vi "MPU_Stick_Event_Counter.vi"(6 "Initialize ?":bool, 8 "error in (no error)":errorcluster, 9 "Event Name":string, 10 "Event count limits":i32[](array[numeric]), 11 "Event names":string[](array[string])) -> (0 "error out":errorcluster, 2 "Event occured":bool, 3 "Events":T1[](array[typedef]))   [LabVIEW 2017]
uses:
  Controls/MPU_Stick_Event.ctl
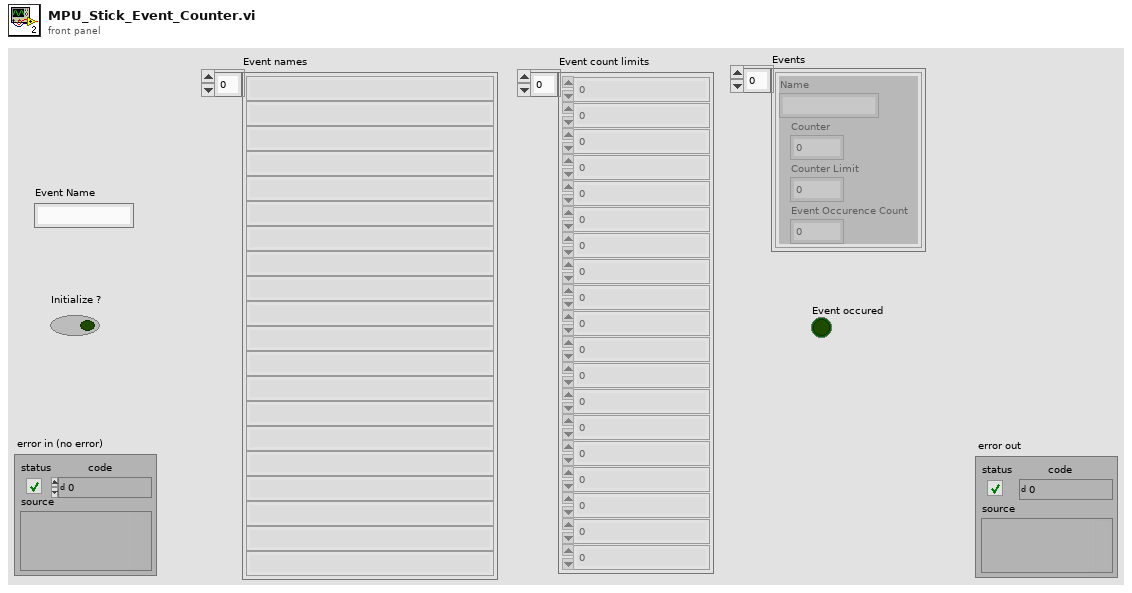
[diagram p1: front panel]
types:
  T1 = typedef "MPU_Stick_Event.ctl" = cluster{"Name":string, "Counter":i32, "Counter Limit":i32, "Event Occurence Count":i32}
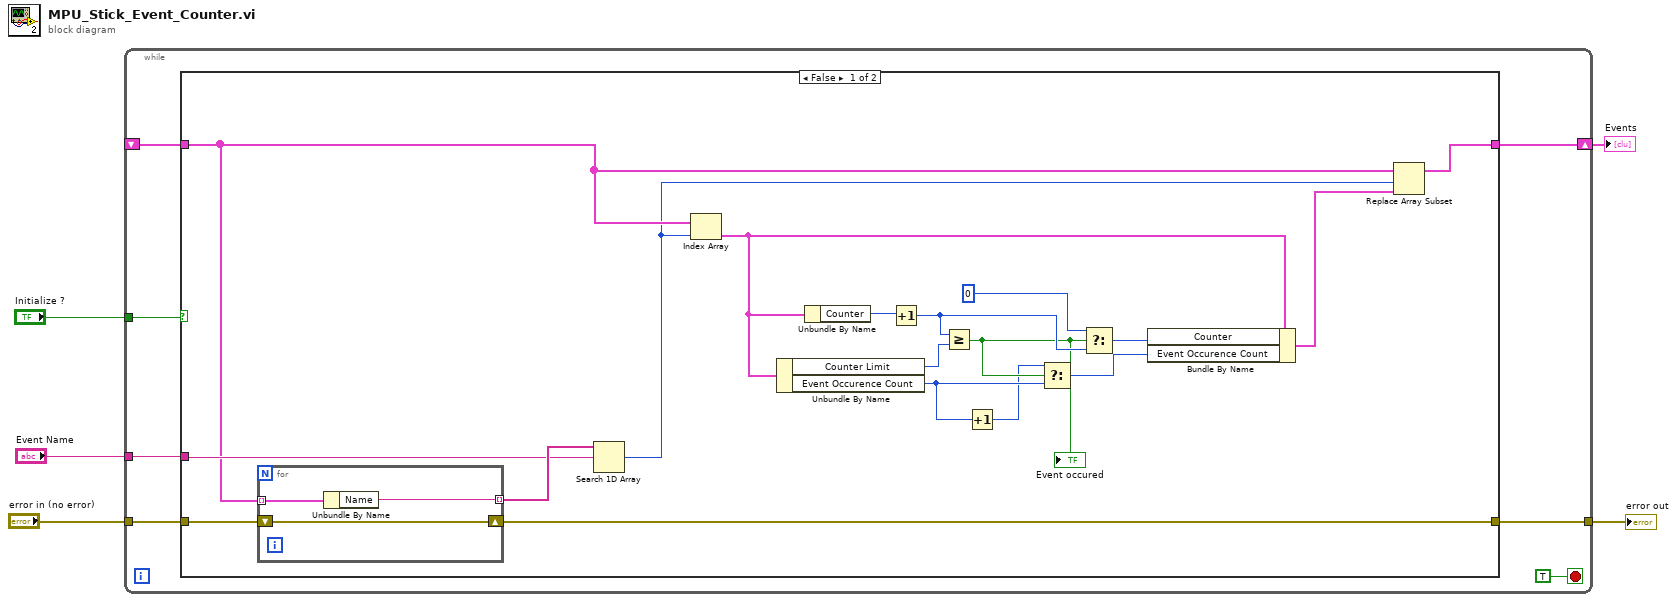
[diagram p0: block diagram]
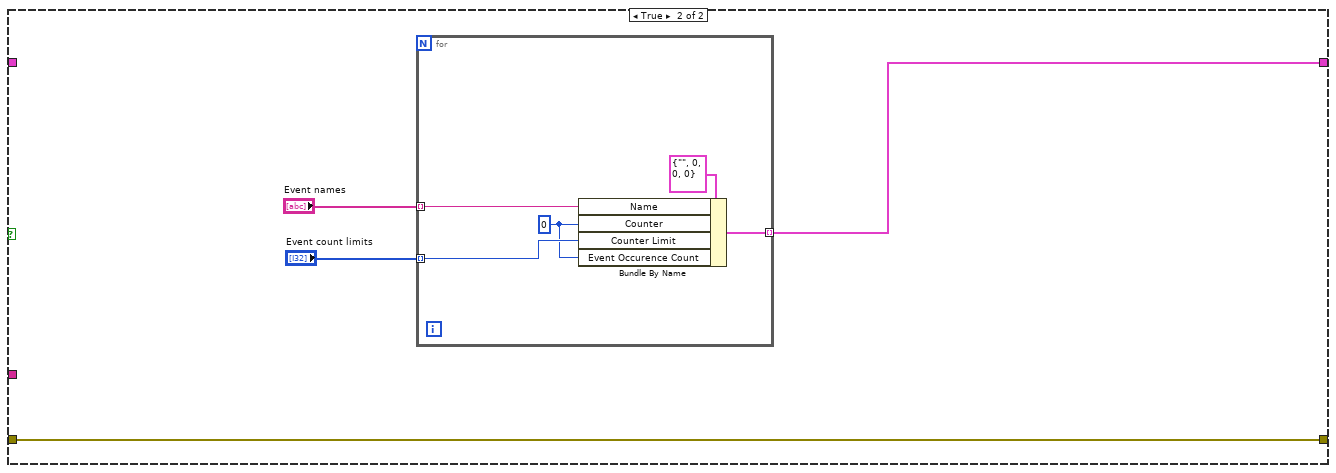
[diagram p2: hidden frame]
diagram:
  n1 = while {
    tunnel: "error in (no error)" -> [w11]
    tunnel: [w10] -> w4
    tunnel: "Initialize ?" -> [w9]
    shift-right: [w8] -> w1
    shift-left: _ -> [w7]
    tunnel: "Event Name" -> [w6]
    stop <- TRUE stop-if-true
    n2 = case shown="False" w9 {
      tunnel: w11 -> [w30 w37]
      tunnel: [w21 w37] -> w10
      tunnel: [w17 w34] -> w8
      tunnel: w7 -> [w20 _]
      tunnel: w6 -> [w28 _]
      frame False {
        n3 = for {
          shift-right: [w33] -> w21
          shift-left: w30 -> [w33]
          tunnel: w20 -> [w32] mode=indexing
          tunnel: [w31] -> w29 mode=indexing
          n4 = Unbundle By Name(w32) -> ("Name"=w31:string)
        }
        n5 = Search 1D Array(1D array=w29, element=w28) -> (index of element=w19:i32)  [unwired: 1 in]
        n6 = Index Array(array=w20, index=w19) -> (element=w23:T1)
        n7 = Unbundle By Name(w23) -> ("Counter Limit"=w26:i32, "Event Occurence Count"=w14:i32)
        n8 = Unbundle By Name(w23) -> ("Counter"=w27:i32)
        n9 = Increment(x=w27) -> (x+1=w25:i32)
        n10 = Greater Or Equal?(x=w25, y=w26) -> (x >= y?=w15:bool)
        "Event occured" <- w15
        n11 = Increment(x=w14) -> (x+1=w13:i32)
        n12 = Select(t=w13, s=w15, f=w14) -> (s? t:f=w16:i32)
        n13 = Select(t=0, s=w15, f=w25) -> (s? t:f=w22:i32)
        n14 = Bundle By Name(cluster=w23, "Counter"=w22, "Event Occurence Count"=w16) -> (w18:T1)
        n15 = Replace Array Subset(array=w20, new element=w18, index=w19) -> (w17:T1[])
      }
      frame True {
        n16 = for {
          tunnel: "Event names" -> [w41] mode=indexing
          tunnel: "Event count limits" -> [w40] mode=indexing
          tunnel: [w38] -> w34 mode=indexing
          w39 = 0 ("Counter")
          n17 = Bundle By Name(cluster=T1 {"Name"="", "Counter"=0, "Counter Limit"=0, "Event Occurence Count"=0} ("Event"), "Name"=w41, "Counter"=w39, "Counter Limit"=w40, "Event Occurence Count"=w39) -> (w38:T1)
        }
      }
    }
  }
  "error out" <- w4
  "Events" <- w1
